vi "Write Close.vi"(0 "FlexChannel":T1) -> ()   [LabVIEW 2020, in "Flex.lvlib"]
doc: "Closes the channel. Performs no other action and when called, immediately stops channel communication. All reader endpoints will be able to see the closed status of the channel and events for the channel will have 1 last event generated where the Closed item will be set to True."
uses:
  Flex.lvlib
  ))Channel.ctl
  Element.ctl
  ChannelOp.ctl
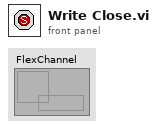
[diagram p1: front panel]
types:
  T1 = typedef "Flex.lvlib/))Channel.ctl" = refnum<queue>
  T2 = typedef "Flex.lvlib/ChannelOp.ctl" = enum16{"Get Refs", "Init", "Close", "Probe", "New Queue", "Remove Queue", "New Event"}
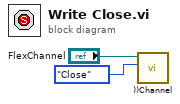
[diagram p0: block diagram]
diagram:
  n1 = call "))Channel.vi"("channelOp"=ChannelOp."Close", "channel in"="FlexChannel") -> ()  [unwired: 5 in, 5 out]
